vi "字符键盘.vi"(11 "Old String":string) -> (3 "String":string)   [LabVIEW 2016]
uses:
  <vilib>/Utility/miscctls.llb/LVPointTypeDef.ctl
panel:
  in  "^":bool
  in  "$":bool
  in  "!":bool
  in  "~":bool
  in  "%":bool
  in  "&":bool
  in  "@":bool
  in  "_":bool
  in  "#":bool
  in  "大小写":bool
  in  "Z":bool
  in  "Y":bool
  in  "X":bool
  in  "W":bool
  in  "V":bool
  in  "U":bool
  in  "T":bool
  in  "S":bool
  in  "R":bool
  in  "Q":bool
  in  "P":bool
  in  "O":bool
  in  "N":bool
  in  "M":bool
  in  "L":bool
  in  "K":bool
  in  "J":bool
  in  "I":bool
  in  "H":bool
  in  "G":bool
  in  "F":bool
  in  "E":bool
  in  "D":bool
  in  "C":bool
  in  "B":bool
  in  "A":bool
  in  ",":bool
  in  "Cancel":bool
  in  "OK":bool
  in  "Clear":bool
  in  "BackSpace":bool
  in  "Point":bool
  in  "Zero":bool
  in  "Nine":bool
  in  "Eight":bool
  in  "Seven":bool
  in  "Six":bool
  in  "Five":bool
  in  "Four":bool
  in  "Three":bool
  in  "Two":bool
  in  "One":bool
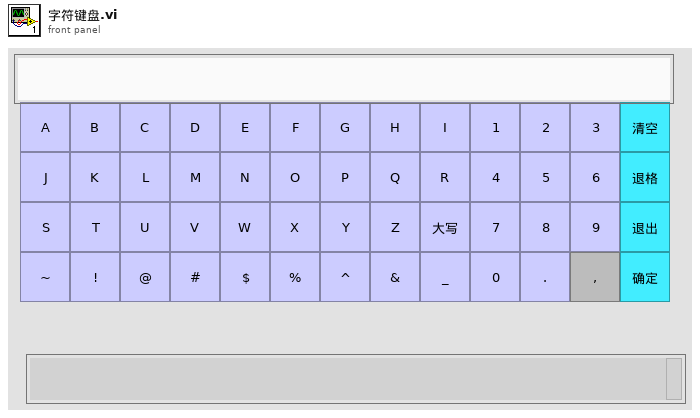
[diagram p1: front panel]
types:
  T1 = typedef "LVPointTypeDef.ctl" = cluster{"Horizontal":i16, "Vertical":i16}
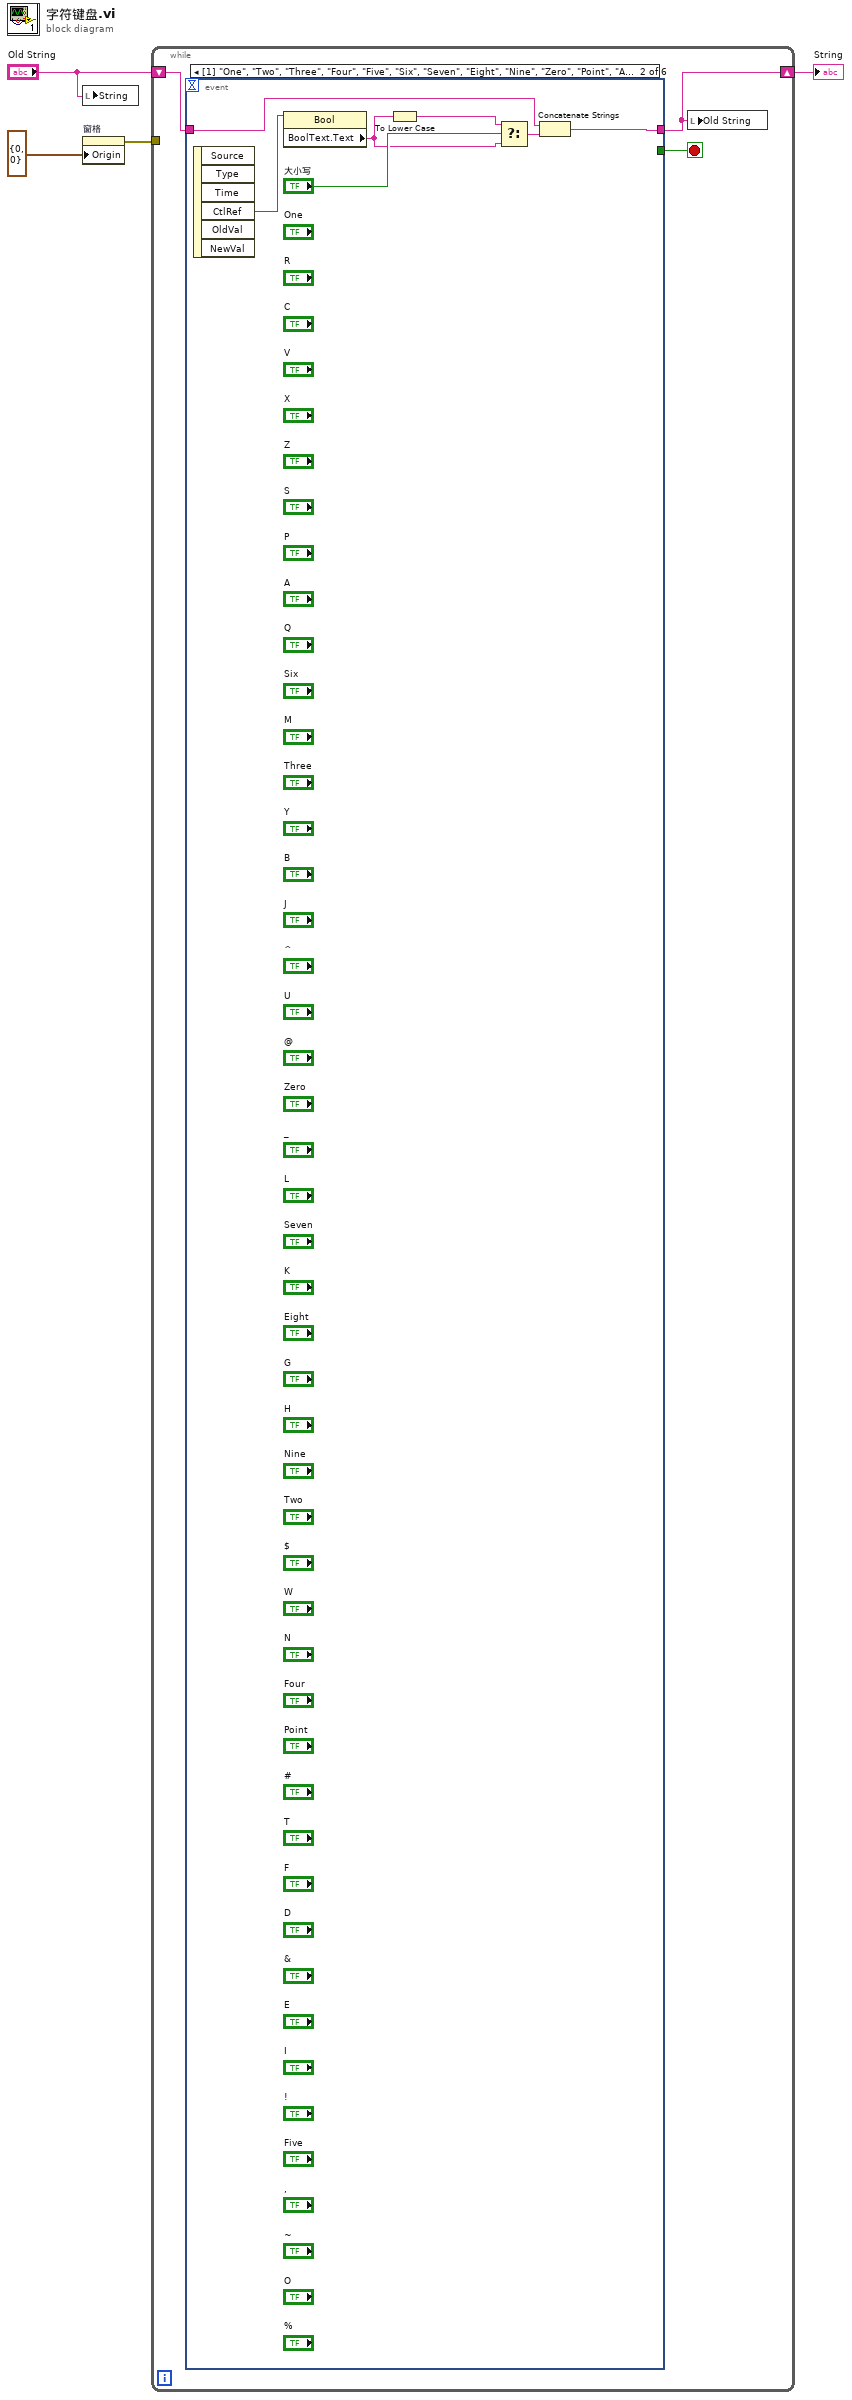
[diagram p0: block diagram]
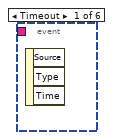
[diagram p2: hidden frame]
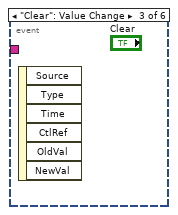
[diagram p3: hidden frame]
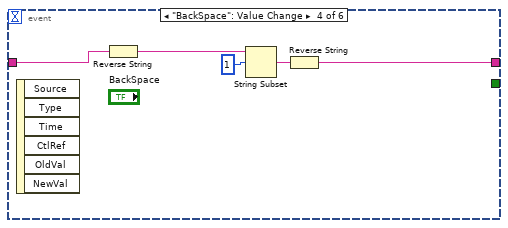
[diagram p4: hidden frame]
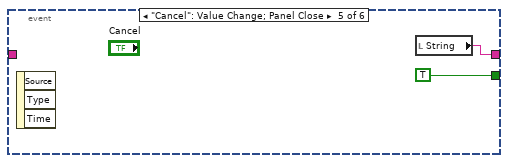
[diagram p5: hidden frame]
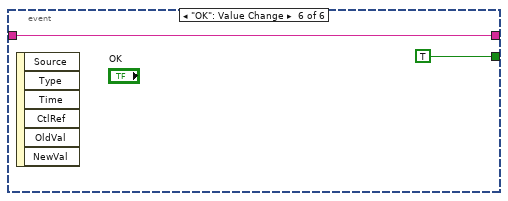
[diagram p6: hidden frame]
diagram:
  n1 = local write "String"("Old String") -> ()
  n2 = property on="窗格" class="Pane"("Origin"=T1 {"Horizontal"=0, "Vertical"=0} ("原点")) -> (error out=w2:errorcluster)  [unwired: 2 in, 1 out]
  n3 = while {
    shift-right: [w5] -> w1
    shift-left: "Old String" -> [w7]
    tunnel: w2 -> [_]
    stop <- w6 stop-if-true
    n4 = event shown="[1] \"One\", \"Two\", \"Three\", \"Four\", \"Five\", \"Six\", \"Seven\", \"Eight\", \"Nine\", \"Zero\", \"Point\", \"A\", \"B\", \"C\", \"D\", \"E\", \"F\", \"G\", \"H\", \"I\", \"J\", \"K\", \"L\", \"M\", \"N\", \"O\", \"P\", \"Q\", \"R\", \"S\", \"T\", \"U\", \"V\", \"W\", \"X\", \"Y\", \"Z\", \"#\", \"_\", \"@\", \"&\", \"%\", \"~\", \"!\", \"$\", \"^\", \",\": 值改变" {
      selector: _ -> [_ _ _ _ _ _]
      dyn-events: _ -> [_ _ _ _ _ _]
      timeout: _ -> [_ _ _ _ _ _]
      tunnel: w7 -> [_ w13 _ w18 _ w23]
      tunnel: [_ w12 _ w15 w21 w23] -> w5
      tunnel: [_ _ _ _ TRUE TRUE] -> w6
      event Timeout {
        n5 = event-data() -> ()  [unwired: 1 in, 3 out]
      }
      event "One", "Two", "Three", "Four", "Five", "Six", "Seven", "Eight", "Nine", "Zero", "Point", "A", "B", "C", "D", "E", "F", "G", "H", "I", "J", "K", "L", "M", "N", "O", "P", "Q", "R", "S", "T", "U", "V", "W", "X", "Y", "Z", "#", "_", "@", "&", "%", "~", "!", "$", "^", ",": Value Change {
        n6 = event-data() -> ("CtlRef"=w14:refnum<vi>)  [unwired: 1 in, 5 out]
        n7 = property class="Bool"(reference=w14) -> ("BoolText.Text"=w8:string)  [unwired: 1 in, 2 out]
        n8 = To Lower Case(string=w8) -> (all lower case string=w9:string)
        n9 = Select(t=w9, s="大小写", f=w8) -> (s? t:f=w10:string)
        n10 = Concatenate Strings(w13, w10) -> (w12:string)
      }
      event "Clear": Value Change {
        n11 = event-data() -> ()  [unwired: 1 in, 6 out]
      }
      event "BackSpace": Value Change {
        n12 = event-data() -> ()  [unwired: 1 in, 6 out]
        n13 = Reverse String(1:w18) -> (0:w17:string)
        n14 = String Subset(string=w17, offset (0)=1 ("偏移量(0)")) -> (substring=w16:string)  [unwired: 1 in]
        n15 = Reverse String(1:w16) -> (0:w15:string)
      }
      event "Cancel": Value Change; Panel Close {
        n16 = event-data() -> ()  [unwired: 1 in, 3 out]
        n17 = local read "String"() -> (w21:string)
      }
      event "OK": Value Change {
        n18 = event-data() -> ()  [unwired: 1 in, 6 out]
      }
    }
    n19 = local write "Old String"(w5) -> ()
  }
  "String" <- w1
